vi "Periodic Tasks.vi"(8 "Error In":errorcluster) -> ()   [LabVIEW 2018]
doc: "This VI runs in parallel to other tasks. It can contain as many user-defined periodic loops as you need. These can carry out PID or other sorts of timed response."
uses:
  <vilib>/Rock Robotics/WPI/Solenoid/WPI_SolenoidValue.ctl
  <vilib>/Rock Robotics/WPI/ThirdParty/Phoenix-LabVIEW/Motor Controller/Controls/CTRE_Phoenix_MotorControl_ControlMode.ctl
  <vilib>/Rock Robotics/WPI/Utilities/WPI_GetSetVariantRefNum.vi
  Global 1.vi
  <vilib>/Rock Robotics/Network Tables/NT Write Boolean.vi
  <vilib>/Rock Robotics/Network Tables/NT Write Number.vi
  <vilib>/Rock Robotics/WPI/Solenoid/WPI_SolenoidSetEnum.vi
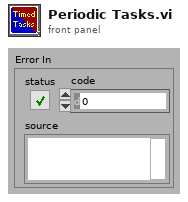
[diagram p1: front panel]
types:
  T1 = typedef "WPI_SwitchDevRef.ctl" = cluster{"DevStatus":errorcluster, "DIO Channel":T2, "CntIndex":T3, "Normally Closed":bool}
  T2 = typedef "FPGA_DIOChannel.ctl" = enum8{"DIO 0", "DIO 1", "DIO 2", "DIO 3", "DIO 4", "DIO 5", "DIO 6", "DIO 7", "DIO 8", "DIO 9", "DIO MXP 0", "DIO MXP 1", "DIO MXP 2", "DIO MXP 3", "DIO MXP 4", "DIO MXP 5", "DIO MXP 6", "DIO MXP 7", "DIO MXP 8", "DIO MXP 9", "DIO MXP 10", "DIO MXP 11", "DIO MXP 12", "DIO MXP 13", "DIO MXP 14", "DIO MXP 15", "SPI Port CS1", "SPI Port CS2", "SPI Port CS3", "SPI Port MISO", "SPI Port MOSI", "Invalid"}
  T3 = typedef "FPGA_CounterCtrSystemIndex.ctl" = enum8{"Ctr 0", "Ctr 1", "Ctr 2", "Ctr 3", "Ctr 4", "Ctr 5", "Ctr 6", "Ctr 7", "Invalid"}
  T4 = typedef "WPI_MotorControlDeviceRef.ctl" = cluster{"DeviceStatus":errorcluster, "Type":T5, "PWM":cluster{"PWM Channel":T6, "DeadBand":T7}, "CAN":cluster{"Device Number":u8, "SetOutput VI Ref":variant, "GetOutput VI Ref":variant, "Enable VI Ref":variant, "Disable VI Ref":variant, "Data":variant}, "Invert":bool, "DIO PWM":cluster{"PWM \"Enable\" Channel":T6, "DIOChannel":T2, "PWM Rate":dbl}}
  T5 = typedef "WPI_MotorControlType.ctl" = enum16{"PWM", "CAN", "DIO PWM"}
  T6 = typedef "FPGA_DIOPWMChannel.ctl" = enum8{"PWM 0", "PWM 1", "PWM 2", "PWM 3", "PWM 4", "PWM 5", "PWM 6", "PWM 7", "PWM 8", "PWM 9", "PWM MXP 0", "PWM MXP 1", "PWM MXP 2", "PWM MXP 3", "PWM MXP 4", "PWM MXP 5", "PWM MXP 6", "PWM MXP 7", "PWM MXP 8", "PWM MXP 9", "Invalid"}
  T7 = typedef "WPI_PWMDeadband.ctl" = cluster{"Name":string, "maxPositivePwm":i32, "minPositivePwm":i32, "centerPwm":i32, "maxNegativePwm":i32, "minNegativePwm":i32, "angularRange":u16}
  T8 = typedef "WPI_JoystickDevRef.ctl" = cluster{"Device":T9}
  T9 = typedef "WPI_JoystickDeviceEnum.ctl" = enum16{"USB 0", "USB 1", "USB 2", "USB 3", "USB 4", "USB 5"}
  T10 = typedef "CTRE_Phoenix_MotorControl_ControlMode.ctl" = u16
  T11 = typedef "WPI_SolenoidDevRef.ctl" = cluster{"DevStatus":errorcluster, "Pneumatics Control Module":u8, "Forward Solenoid Channel":T12, "Reverse Solenoid Channel":T12}
  T12 = typedef "WPI_SolenoidChannel.ctl" = enum8{"Solenoid 0", "Solenoid 1", "Solenoid 2", "Solenoid 3", "Solenoid 4", "Solenoid 5", "Solenoid 6", "Solenoid 7", "Invalid"}
  T13 = typedef "WPI_SolenoidValue.ctl" = enum16{"Off", "On", "Forward", "Reverse"}
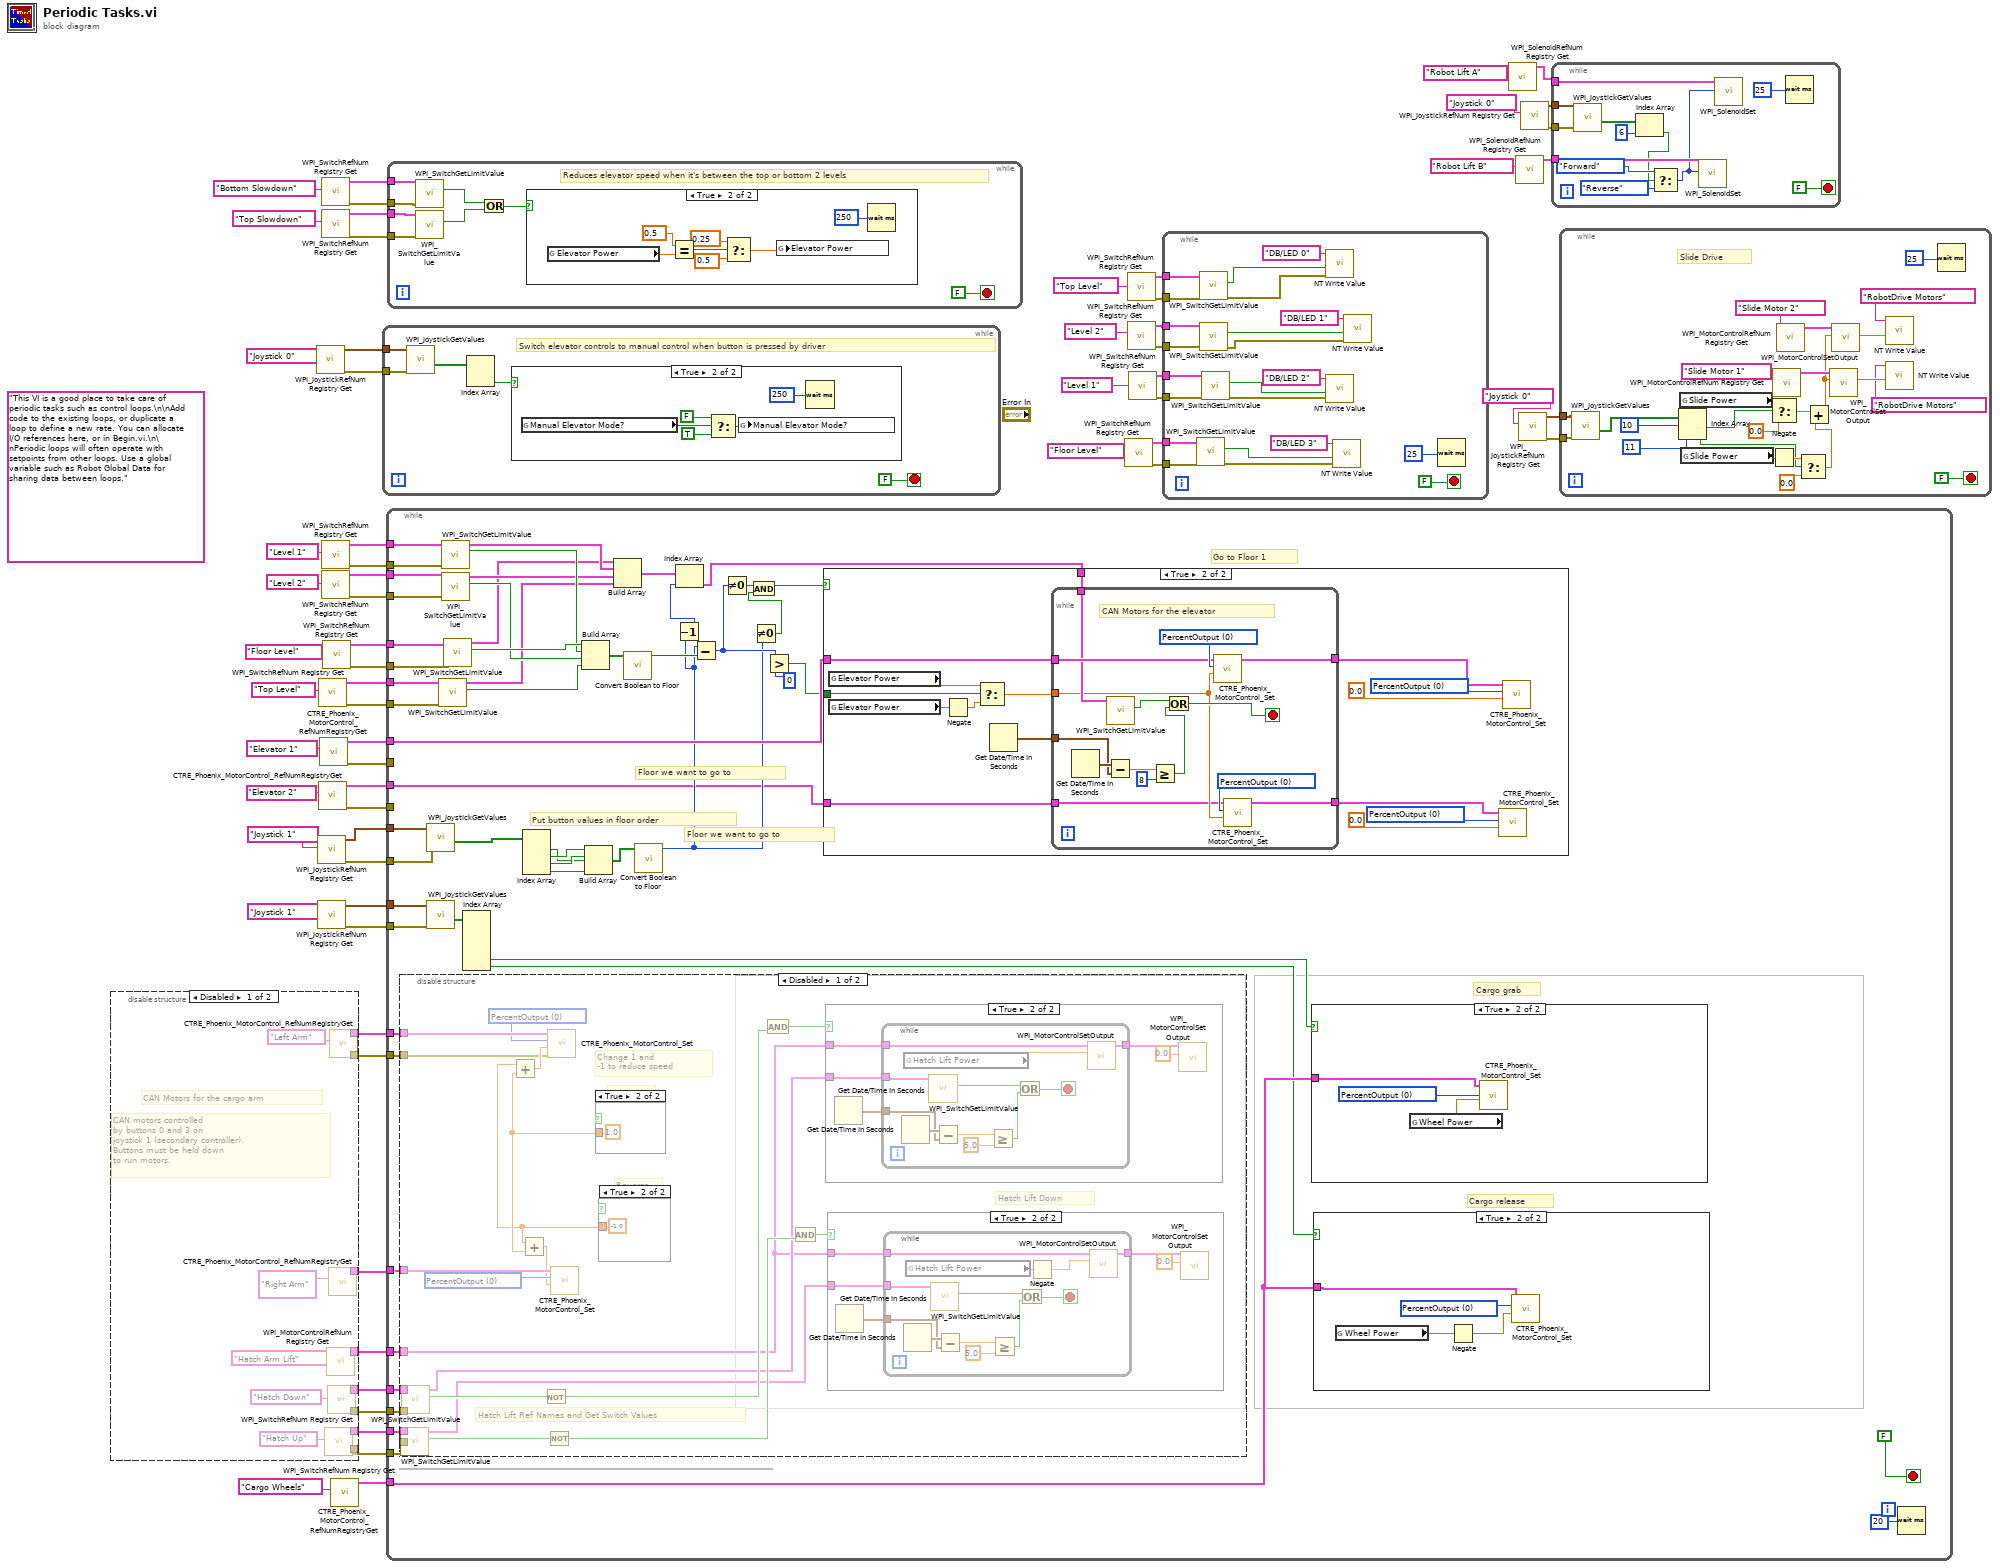
[diagram p0: block diagram]
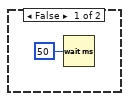
[diagram p3: hidden frame]
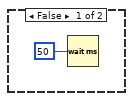
[diagram p4: hidden frame]
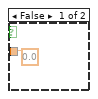
[diagram p7: hidden frame]
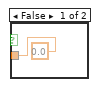
[diagram p8: hidden frame]
diagram:
  (unwired) "This VI is a good place to take care of periodic tasks such as control loops.\n\nAdd code to the existing loops, or duplicate a loop to define a new rate. You can allocate I/O references here, or in Begin.vi.\n\nPeriodic loops will often operate with setpoints from other loops. Use a global variable such as Robot Global Data for sharing data between loops."
  n1 = disable-structure shown="Disabled" {
    disable-tunnel: [w78 _] -> w63
    disable-tunnel: [w77 _] -> w62
    disable-tunnel: [w74 _] -> w46
    disable-tunnel: [w70 _] -> w33
    disable-tunnel: [w69 _] -> w32
    disable-tunnel: [w68 _] -> w31
    disable-tunnel: [w67 _] -> w30
    disable-tunnel: [w66 _] -> w29
    frame Disabled {
      # "CAN Motors for the cargo arm"
      # "CAN motors controlled\nby buttons 0 and 3 on \njoystick 1 (secondary controller).\nButtons must be held down\nto run motors."
      n2 = call <vilib>:"WPI_SwitchRefNum Registry Get.vi"("refnum name"="Hatch Up") -> ("error out"=w69:errorcluster, "SwitchDevRef"=w70:T1)  [unwired: 9 in]
      n3 = call <vilib>:"WPI_MotorControlRefNum Registry Get.vi"("refnum name"="Hatch Arm Lift") -> ("MotorControlDevRef"=w66:T4)  [unwired: 9 in, 1 out]
      n4 = call <vilib>:"WPI_SwitchRefNum Registry Get.vi"("refnum name"="Hatch Down") -> ("error out"=w68:errorcluster, "SwitchDevRef"=w67:T1)  [unwired: 9 in]
      n5 = call <vilib>:"CTRE_Phoenix_MotorControl_RefNumRegistryGet.vi"("refnum name"="Right Arm") -> ("PhoenixMotorControlDevRef"=w77:T4)  [unwired: 9 in, 1 out]
      n6 = call <vilib>:"CTRE_Phoenix_MotorControl_RefNumRegistryGet.vi"("refnum name"="Left Arm") -> ("error out"=w74:errorcluster, "PhoenixMotorControlDevRef"=w78:T4)  [unwired: 9 in]
    }
    frame Enabled {
    }
  }
  n7 = call <vilib>:"WPI_JoystickRefNum Registry Get.vi"("refnum name"="Joystick 0") -> ("error out"=w53:errorcluster, "JoystickDevRef"=w54:T8)  [unwired: 9 in]
  n8 = call <vilib>:"WPI_JoystickRefNum Registry Get.vi"("refnum name"="Joystick 1") -> ("error out"=w47:errorcluster, "JoystickDevRef"=w58:T8)  [unwired: 9 in]
  n9 = call <vilib>:"WPI_JoystickRefNum Registry Get.vi"("refnum name"="Joystick 1") -> ("error out"=w52:errorcluster, "JoystickDevRef"=w60:T8)  [unwired: 9 in]
  n10 = call <vilib>:"WPI_SwitchRefNum Registry Get.vi"("refnum name"="Top Level") -> ("error out"=w51:errorcluster, "SwitchDevRef"=w61:T1)  [unwired: 9 in]
  n11 = call <vilib>:"CTRE_Phoenix_MotorControl_RefNumRegistryGet.vi"("refnum name"="Elevator 2") -> ("error out"=w14:errorcluster, "PhoenixMotorControlDevRef"=w21:T4)  [unwired: 9 in]
  n12 = call <vilib>:"CTRE_Phoenix_MotorControl_RefNumRegistryGet.vi"("refnum name"="Elevator 1") -> ("error out"=w13:errorcluster, "PhoenixMotorControlDevRef"=w59:T4)  [unwired: 9 in]
  n13 = call <vilib>:"WPI_SwitchRefNum Registry Get.vi"("refnum name"="Bottom Slowdown") -> ("error out"=w15:errorcluster, "SwitchDevRef"=w18:T1)  [unwired: 9 in]
  n14 = call <vilib>:"WPI_SwitchRefNum Registry Get.vi"("refnum name"="Top Slowdown") -> ("error out"=w16:errorcluster, "SwitchDevRef"=w17:T1)  [unwired: 9 in]
  n15 = call <vilib>:"WPI_SwitchRefNum Registry Get.vi"("refnum name"="Level 1") -> ("error out"=w48:errorcluster, "SwitchDevRef"=w65:T1)  [unwired: 9 in]
  n16 = call <vilib>:"WPI_SwitchRefNum Registry Get.vi"("refnum name"="Level 2") -> ("error out"=w49:errorcluster, "SwitchDevRef"=w64:T1)  [unwired: 9 in]
  n17 = call <vilib>:"WPI_SwitchRefNum Registry Get.vi"("refnum name"="Floor Level") -> ("error out"=w50:errorcluster, "SwitchDevRef"=w57:T1)  [unwired: 9 in]
  n18 = call <vilib>:"CTRE_Phoenix_MotorControl_RefNumRegistryGet.vi"("refnum name"="Cargo Wheels") -> ("PhoenixMotorControlDevRef"=w3:T4)  [unwired: 9 in, 1 out]
  n19 = while {
    tunnel: w54 -> [w83]
    tunnel: w53 -> [w82]
    stop <- FALSE stop-if-true
    # "Switch elevator controls to manual control when button is pressed by driver"
    n20 = call <vilib>:"WPI_JoystickGetValues.vi"("error in (no error)"=w82, "JoystickDevRef"=w83) -> ("Buttons"=w81:bool[])  [unwired: 5 in, 4 out]
    n21 = Index Array(array=w81) -> (element #2=w80:bool)  [unwired: 2 in, 1 out]
    n22 = case shown="True" w80 {
      frame False {
        n23 = Wait (ms)(milliseconds to wait=u32 50) -> ()  [unwired: 1 out]
      }
      frame True {
        n24 = global read "Global 1.vi" "Manual Elevator Mode?"() -> (w89:bool)
        n25 = Select(t=FALSE, s=w89, f=TRUE) -> (s? t:f=w88:bool)
        n26 = global write "Global 1.vi" "Manual Elevator Mode?"(w88) -> ()
        n27 = Wait (ms)(milliseconds to wait=u32 250) -> ()  [unwired: 1 out]
      }
    }
  }
  n28 = while {
    tunnel: w65 -> [w141]
    tunnel: w64 -> [w140]
    tunnel: w63 -> [w139]
    tunnel: w62 -> [w138]
    tunnel: w61 -> [w137]
    tunnel: w60 -> [w136]
    tunnel: w59 -> [w133]
    tunnel: w58 -> [w135]
    tunnel: w57 -> [w134]
    tunnel: w52 -> [w131]
    tunnel: w51 -> [w130]
    tunnel: w50 -> [w129]
    tunnel: w49 -> [w128]
    tunnel: w48 -> [w127]
    tunnel: w47 -> [w126]
    tunnel: w46 -> [w125]
    tunnel: w33 -> [w124]
    tunnel: w32 -> [w123]
    tunnel: w31 -> [w122]
    tunnel: w30 -> [w121]
    tunnel: w29 -> [w120]
    tunnel: w3 -> [w119]
    tunnel: w21 -> [w98]
    tunnel: w14 -> [_]
    tunnel: w13 -> [_]
    stop <- FALSE stop-if-true
    # "Put button values in floor order"
    # "Floor we want to go to"
    # "Floor we want to go to"
    # "Go to Floor 1"
    # "Cargo release"
    # "Cargo grab"
    n29 = disable-structure shown="Disabled" {
      disable-tunnel: w139 -> [w165 _]
      disable-tunnel: w138 -> [w164 _]
      disable-tunnel: w125 -> [w157 _]
      disable-tunnel: w124 -> [w156 _]
      disable-tunnel: w123 -> [w155 _]
      disable-tunnel: w122 -> [w154 _]
      disable-tunnel: w121 -> [w153 _]
      disable-tunnel: w120 -> [w145 _]
      frame Disabled {
        w161 = T10 0 items=["PercentOutput"=0, "Position"=1, "Velocity"=2, "Current"=3, "Follower"=5, "MotionProfile"=6, "MotionMagic"=7, "MotionProfileArc"=10, "Disabled"=15] ("Control Mode")
        w163 = T10 0 items=["PercentOutput"=0, "Position"=1, "Velocity"=2, "Current"=3, "Follower"=5, "MotionProfile"=6, "MotionMagic"=7, "MotionProfileArc"=10, "Disabled"=15] ("Control Mode")
        # "Hatch Lift Ref Names and Get Switch Values"
        # "Hatch Lift Down"
        # "Change 1 and\n-1 to reduce speed"
        # "Forward"
        # "Reverse"
        n30 = call <vilib>:"WPI_SwitchGetLimitValue.vi"("error in (no error)"=w155, "SwitchDevRef"=w156) -> ("Switch Pressed"=w152:bool, "SwitchDevRef"=w144:T1)  [unwired: 7 in, 1 out]
        n31 = call <vilib>:"WPI_SwitchGetLimitValue.vi"("error in (no error)"=w154, "SwitchDevRef"=w153) -> ("Switch Pressed"=w150:bool, "SwitchDevRef"=w146:T1)  [unwired: 7 in, 1 out]
        n32 = Not(x=w150) -> (.not. x?=w149:bool)
        n33 = Not(x=w152) -> (.not. x?=w148:bool)
        n34 = case shown="True" {
          selector: _ -> [_ _]
          tunnel: [0.0 1.0] -> w159
          frame False {
          }
          frame True {
          }
        }
        n35 = case shown="True" {
          selector: _ -> [_ _]
          tunnel: [0.0 -1.0] -> w158
          frame False {
          }
          frame True {
          }
        }
        n36 = Add(x=w158, y=w159) -> (x+y=w162:dbl)
        n37 = Add(x=w158, y=w159) -> (x+y=w160:dbl)
        n38 = call <vilib>:"CTRE_Phoenix_MotorControl_Set.vi"("error in (no error)"=w157, "Output"=w162, "Control Mode"=w163, "PhoenixMotorControlDevRef"=w165) -> ()  [unwired: 6 in, 2 out]
        n39 = call <vilib>:"CTRE_Phoenix_MotorControl_Set.vi"("Output"=w160, "Control Mode"=w161, "PhoenixMotorControlDevRef"=w164) -> ()  [unwired: 7 in, 2 out]
        n40 = And(y=w149) -> (x .and. y?=w151:bool)  [unwired: 1 in]
        n41 = And(y=w148) -> (x .and. y?=w147:bool)  [unwired: 1 in]
        n42 = case shown="True" w151 {
          tunnel: w146 -> [_ w187]
          tunnel: w145 -> [_ w186]
          frame False {
          }
          frame True {
            n43 = Get Date/Time In Seconds() -> (seconds since 1Jan1904=w185:timestamp)
            n44 = while {
              tunnel: w187 -> [w198]
              tunnel: w186 -> [w197]
              tunnel: w185 -> [w193]
              tunnel: [w189] -> w184
              stop <- w192 stop-if-true
              n45 = Get Date/Time In Seconds() -> (seconds since 1Jan1904=w194:timestamp)
              n46 = global read "Global 1.vi" "Hatch Lift Power"() -> (w196:dbl)
              n47 = call <vilib>:"WPI_SwitchGetLimitValue.vi"("SwitchDevRef"=w198) -> ("Switch Pressed"=w191:bool)  [unwired: 8 in, 2 out]
              n48 = Subtract(x=w194, y=w193) -> (x-y=w195:dbl)
              n49 = Greater Or Equal?(x=w195, y=5.0) -> (x >= y?=w190:bool)
              n50 = Or(x=w191, y=w190) -> (x .or. y?=w192:bool)
              n51 = call <vilib>:"WPI_MotorControlSetOutput.vi"("Output"=w196, "MotorControlDevRef"=w197) -> ("MotorControlDevRef"=w189:T4)  [unwired: 7 in, 2 out]
            }
            n52 = call <vilib>:"WPI_MotorControlSetOutput.vi"("Output"=0.0, "MotorControlDevRef"=w184) -> ()  [unwired: 7 in, 3 out]
          }
        }
        n53 = case shown="True" w147 {
          tunnel: w144 -> [_ w170]
          tunnel: w145 -> [_ w169]
          frame False {
          }
          frame True {
            n54 = Get Date/Time In Seconds() -> (seconds since 1Jan1904=w168:timestamp)
            n55 = while {
              tunnel: w170 -> [w182]
              tunnel: w169 -> [w181]
              tunnel: w168 -> [w177]
              tunnel: [w173] -> w167
              stop <- w176 stop-if-true
              n56 = Get Date/Time In Seconds() -> (seconds since 1Jan1904=w178:timestamp)
              n57 = global read "Global 1.vi" "Hatch Lift Power"() -> (w180:dbl)
              n58 = call <vilib>:"WPI_SwitchGetLimitValue.vi"("SwitchDevRef"=w182) -> ("Switch Pressed"=w175:bool)  [unwired: 8 in, 2 out]
              n59 = Subtract(x=w178, y=w177) -> (x-y=w179:dbl)
              n60 = Greater Or Equal?(x=w179, y=5.0) -> (x >= y?=w174:bool)
              n61 = Or(x=w175, y=w174) -> (x .or. y?=w176:bool)
              n62 = Negate(x=w180) -> (-x=w172:dbl)
              n63 = call <vilib>:"WPI_MotorControlSetOutput.vi"("Output"=w172, "MotorControlDevRef"=w181) -> ("MotorControlDevRef"=w173:T4)  [unwired: 7 in, 2 out]
            }
            n64 = call <vilib>:"WPI_MotorControlSetOutput.vi"("Output"=0.0, "MotorControlDevRef"=w167) -> ()  [unwired: 7 in, 3 out]
          }
        }
      }
      frame Enabled {
      }
    }
    n65 = call <vilib>:"WPI_JoystickGetValues.vi"("error in (no error)"=w126, "JoystickDevRef"=w135) -> ("Buttons"=w97:bool[])  [unwired: 5 in, 4 out]
    n66 = call <vilib>:"WPI_JoystickGetValues.vi"("error in (no error)"=w131, "JoystickDevRef"=w136) -> ("Buttons"=w132:bool[])  [unwired: 5 in, 4 out]
    n67 = call <vilib>:"WPI_SwitchGetLimitValue.vi"("error in (no error)"=w130, "SwitchDevRef"=w137) -> ("Switch Pressed"=w117:bool, "SwitchDevRef"=w106:T1)  [unwired: 7 in, 1 out]
    n68 = call <vilib>:"WPI_SwitchGetLimitValue.vi"("error in (no error)"=w127, "SwitchDevRef"=w141) -> ("Switch Pressed"=w115:bool, "SwitchDevRef"=w108:T1)  [unwired: 7 in, 1 out]
    n69 = call <vilib>:"WPI_SwitchGetLimitValue.vi"("error in (no error)"=w128, "SwitchDevRef"=w140) -> ("Switch Pressed"=w114:bool, "SwitchDevRef"=w107:T1)  [unwired: 7 in, 1 out]
    n70 = call <vilib>:"WPI_SwitchGetLimitValue.vi"("error in (no error)"=w129, "SwitchDevRef"=w134) -> ("Switch Pressed"=w116:bool, "SwitchDevRef"=w105:T1)  [unwired: 7 in, 1 out]
    n71 = Index Array(array=w132) -> (element #5=w91:bool, element #6=w90:bool)  [unwired: 6 in, 4 out]
    n72 = Index Array(array=w97) -> (element #1=w94:bool, element #2=w96:bool, element #3=w95:bool, element #4=w93:bool)  [unwired: 4 in]
    n73 = Build Array(w116, w115, w114, w117) -> (w118:bool[])
    n74 = Build Array(w96, w95, w94, w93) -> (w92:bool[])
    n75 = Build Array(w105, w108, w107, w106) -> (w104:T1[])
    n76 = call "Convert Boolean to Floor.vi"("Boolean array"=w118) -> ("Floor Number"=w112:i32)  [unwired: 8 in, 2 out]
    n77 = call "Convert Boolean to Floor.vi"("Boolean array"=w92) -> ("Floor Number"=w100:i32)  [unwired: 8 in, 2 out]
    n78 = Decrement(x=w100) -> (x-1=w102:i32)
    n79 = Index Array(array=w104, index=w102) -> (element=w103:T1)
    n80 = Subtract(x=w100, y=w112) -> (x-y=w111:i32)
    n81 = Not Equal To 0?(x=w111) -> (x != 0?=w113:bool)
    n82 = Not Equal To 0?(x=w100) -> (x != 0?=w99:bool)
    n83 = And(x=w113, y=w99) -> (x .and. y?=w101:bool)
    n84 = Greater?(x=w111, y=0) -> (0:w109:bool)
    n85 = case shown="True" w101 {
      tunnel: w133 -> [_ w217]
      tunnel: w103 -> [_ w213]
      tunnel: w109 -> [_ w210]
      tunnel: w98 -> [_ w203]
      frame False {
      }
      frame True {
        w206 = T10 0 items=["PercentOutput"=0, "Position"=1, "Velocity"=2, "Current"=3, "Follower"=5, "MotionProfile"=6, "MotionMagic"=7, "MotionProfileArc"=10, "Disabled"=15] ("Control Mode")
        w216 = T10 0 items=["PercentOutput"=0, "Position"=1, "Velocity"=2, "Current"=3, "Follower"=5, "MotionProfile"=6, "MotionMagic"=7, "MotionProfileArc"=10, "Disabled"=15] ("Control Mode")
        n86 = global read "Global 1.vi" "Elevator Power"() -> (w209:dbl)
        n87 = global read "Global 1.vi" "Elevator Power"() -> (w207:dbl)
        n88 = Negate(x=w207) -> (-x=w208:dbl)
        n89 = Select(t=w209, s=w210, f=w208) -> (s? t:f=w212:dbl)
        n90 = Get Date/Time In Seconds() -> (seconds since 1Jan1904=w211:timestamp)
        n91 = while {
          tunnel: w217 -> [w231]
          tunnel: [w230] -> w214
          tunnel: w213 -> [w229]
          tunnel: w212 -> [w221]
          tunnel: w211 -> [w225]
          tunnel: [w219] -> w205
          tunnel: w203 -> [w218]
          stop <- w228 stop-if-true
          w220 = T10 0 items=["PercentOutput"=0, "Position"=1, "Velocity"=2, "Current"=3, "Follower"=5, "MotionProfile"=6, "MotionMagic"=7, "MotionProfileArc"=10, "Disabled"=15] ("Control Mode")
          w232 = T10 0 items=["PercentOutput"=0, "Position"=1, "Velocity"=2, "Current"=3, "Follower"=5, "MotionProfile"=6, "MotionMagic"=7, "MotionProfileArc"=10, "Disabled"=15] ("Control Mode")
          # "CAN Motors for the elevator"
          n92 = Get Date/Time In Seconds() -> (seconds since 1Jan1904=w226:timestamp)
          n93 = call <vilib>:"WPI_SwitchGetLimitValue.vi"("SwitchDevRef"=w229) -> ("Switch Pressed"=w227:bool)  [unwired: 8 in, 2 out]
          n94 = Subtract(x=w226, y=w225) -> (x-y=w223:dbl)
          n95 = Greater Or Equal?(x=w223, y=8) -> (x >= y?=w222:bool)
          n96 = Or(x=w227, y=w222) -> (x .or. y?=w228:bool)
          n97 = call <vilib>:"CTRE_Phoenix_MotorControl_Set.vi"("Output"=w221, "Control Mode"=w232, "PhoenixMotorControlDevRef"=w231) -> ("PhoenixMotorControlDevRef"=w230:T4)  [unwired: 7 in, 1 out]
          n98 = call <vilib>:"CTRE_Phoenix_MotorControl_Set.vi"("Output"=w221, "Control Mode"=w220, "PhoenixMotorControlDevRef"=w218) -> ("PhoenixMotorControlDevRef"=w219:T4)  [unwired: 7 in, 1 out]
        }
        n99 = call <vilib>:"CTRE_Phoenix_MotorControl_Set.vi"("Output"=0.0, "Control Mode"=w206, "PhoenixMotorControlDevRef"=w205) -> ()  [unwired: 7 in, 2 out]
        n100 = call <vilib>:"CTRE_Phoenix_MotorControl_Set.vi"("Output"=0.0, "Control Mode"=w216, "PhoenixMotorControlDevRef"=w214) -> ()  [unwired: 7 in, 2 out]
      }
    }
    n101 = case shown="True" w91 {
      tunnel: w119 -> [_ w237]
      frame False {
      }
      frame True {
        w238 = T10 0 items=["PercentOutput"=0, "Position"=1, "Velocity"=2, "Current"=3, "Follower"=5, "MotionProfile"=6, "MotionMagic"=7, "MotionProfileArc"=10, "Disabled"=15] ("Control Mode")
        n102 = global read "Global 1.vi" "Wheel Power"() -> (w239:dbl)
        n103 = call <vilib>:"CTRE_Phoenix_MotorControl_Set.vi"("Output"=w239, "Control Mode"=w238, "PhoenixMotorControlDevRef"=w237) -> ()  [unwired: 7 in, 2 out]
      }
    }
    n104 = case shown="True" w90 {
      tunnel: w119 -> [_ w235]
      frame False {
      }
      frame True {
        w236 = T10 0 items=["PercentOutput"=0, "Position"=1, "Velocity"=2, "Current"=3, "Follower"=5, "MotionProfile"=6, "MotionMagic"=7, "MotionProfileArc"=10, "Disabled"=15] ("Control Mode")
        n105 = global read "Global 1.vi" "Wheel Power"() -> (w234:dbl)
        n106 = Negate(x=w234) -> (-x=w233:dbl)
        n107 = call <vilib>:"CTRE_Phoenix_MotorControl_Set.vi"("Output"=w233, "Control Mode"=w236, "PhoenixMotorControlDevRef"=w235) -> ()  [unwired: 7 in, 2 out]
      }
    }
    n108 = Wait (ms)(milliseconds to wait=u32 20) -> ()  [unwired: 1 out]
  }
  n109 = while {
    tunnel: w18 -> [w247]
    tunnel: w17 -> [w246]
    tunnel: w16 -> [w245]
    tunnel: w15 -> [w244]
    stop <- FALSE stop-if-true
    # "Reduces elevator speed when it's between the top or bottom 2 levels"
    n110 = call <vilib>:"WPI_SwitchGetLimitValue.vi"("error in (no error)"=w244, "SwitchDevRef"=w247) -> ("Switch Pressed"=w243:bool)  [unwired: 7 in, 2 out]
    n111 = call <vilib>:"WPI_SwitchGetLimitValue.vi"("error in (no error)"=w245, "SwitchDevRef"=w246) -> ("Switch Pressed"=w241:bool)  [unwired: 7 in, 2 out]
    n112 = Or(x=w243, y=w241) -> (x .or. y?=w242:bool)
    n113 = case shown="True" w242 {
      frame False {
        n114 = Wait (ms)(milliseconds to wait=u32 50) -> ()  [unwired: 1 out]
      }
      frame True {
        n115 = global read "Global 1.vi" "Elevator Power"() -> (w255:dbl)
        n116 = Equal?(x=0.5, y=w255) -> (x = y?=w254:bool)
        n117 = Select(t=0.25, s=w254, f=0.5) -> (s? t:f=w250:dbl)
        n118 = global write "Global 1.vi" "Elevator Power"(w250) -> ()
        n119 = Wait (ms)(milliseconds to wait=u32 250) -> ()  [unwired: 1 out]
      }
    }
  }
  n120 = call <vilib>:"WPI_SwitchRefNum Registry Get.vi"("refnum name"="Floor Level") -> ("error out"=w40:errorcluster, "SwitchDevRef"=w39:T1)  [unwired: 9 in]
  n121 = call <vilib>:"WPI_SwitchRefNum Registry Get.vi"("refnum name"="Top Level") -> ("error out"=w44:errorcluster, "SwitchDevRef"=w45:T1)  [unwired: 9 in]
  n122 = call <vilib>:"WPI_SwitchRefNum Registry Get.vi"("refnum name"="Level 2") -> ("error out"=w42:errorcluster, "SwitchDevRef"=w43:T1)  [unwired: 9 in]
  n123 = call <vilib>:"WPI_SwitchRefNum Registry Get.vi"("refnum name"="Level 1") -> ("error out"=w38:errorcluster, "SwitchDevRef"=w41:T1)  [unwired: 9 in]
  n124 = while {
    tunnel: w45 -> [w277]
    tunnel: w44 -> [w276]
    tunnel: w43 -> [w275]
    tunnel: w42 -> [w274]
    tunnel: w41 -> [w273]
    tunnel: w40 -> [w272]
    tunnel: w39 -> [w271]
    tunnel: w38 -> [w270]
    stop <- FALSE stop-if-true
    n125 = call <vilib>:"WPI_SwitchGetLimitValue.vi"("error in (no error)"=w272, "SwitchDevRef"=w271) -> ("error out"=w256:errorcluster, "Switch Pressed"=w262:bool)  [unwired: 7 in, 1 out]
    n126 = call <vilib>:"WPI_SwitchGetLimitValue.vi"("error in (no error)"=w276, "SwitchDevRef"=w277) -> ("error out"=w259:errorcluster, "Switch Pressed"=w268:bool)  [unwired: 7 in, 1 out]
    n127 = call <vilib>:"WPI_SwitchGetLimitValue.vi"("error in (no error)"=w274, "SwitchDevRef"=w275) -> ("error out"=w258:errorcluster, "Switch Pressed"=w266:bool)  [unwired: 7 in, 1 out]
    n128 = call <vilib>:"WPI_SwitchGetLimitValue.vi"("error in (no error)"=w270, "SwitchDevRef"=w273) -> ("error out"=w257:errorcluster, "Switch Pressed"=w264:bool)  [unwired: 7 in, 1 out]
    n129 = call-poly <vilib>:"NT Write Value.vi"("error in"=w259, "Boolean"=w268, "Name"="DB/LED 0") -> ()  [unwired: 8 in, 1 out]
    n130 = call-poly <vilib>:"NT Write Value.vi"("error in"=w257, "Boolean"=w264, "Name"="DB/LED 2") -> ()  [unwired: 8 in, 1 out]
    n131 = call-poly <vilib>:"NT Write Value.vi"("error in"=w256, "Boolean"=w262, "Name"="DB/LED 3") -> ()  [unwired: 8 in, 1 out]
    n132 = call-poly <vilib>:"NT Write Value.vi"("error in"=w258, "Boolean"=w266, "Name"="DB/LED 1") -> ()  [unwired: 8 in, 1 out]
    n133 = Wait (ms)(milliseconds to wait=u32 25 ("millisecond timer value")) -> ()  [unwired: 1 out]
  }
  n134 = call <vilib>:"WPI_SolenoidRefNum Registry Get.vi"("refnum name"="Robot Lift A") -> ("SolenoidDevRef"=w1:T11)  [unwired: 9 in, 1 out]
  n135 = call <vilib>:"WPI_SolenoidRefNum Registry Get.vi"("refnum name"="Robot Lift B") -> ("SolenoidDevRef"=w5:T11)  [unwired: 9 in, 1 out]
  n136 = call <vilib>:"WPI_JoystickRefNum Registry Get.vi"("refnum name"="Joystick 0") -> ("error out"=w10:errorcluster, "JoystickDevRef"=w11:T8)  [unwired: 9 in]
  n137 = call <vilib>:"WPI_JoystickRefNum Registry Get.vi"("refnum name"="Joystick 0") -> ("error out"=w7:errorcluster, "JoystickDevRef"=w8:T8)  [unwired: 9 in]
  n138 = while {
    tunnel: w8 -> [w287]
    tunnel: w7 -> [w286]
    tunnel: w5 -> [w283]
    tunnel: w1 -> [w279]
    stop <- FALSE stop-if-true
    n139 = call <vilib>:"WPI_JoystickGetValues.vi"("error in (no error)"=w286, "JoystickDevRef"=w287) -> ("Buttons"=w285:bool[])  [unwired: 5 in, 4 out]
    n140 = Index Array(array=w285, index=6) -> (element=w280:bool)
    n141 = Select(t=WPI_SolenoidValue."Forward" ("Value"), s=w280, f=WPI_SolenoidValue."Reverse" ("Value")) -> (s? t:f=w278:T13)
    n142 = call-poly <vilib>:"WPI_SolenoidSet.vi"("Value"=w278, "SolenoidDevRef"=w283) -> ()  [unwired: 8 in, 2 out]
    n143 = call-poly <vilib>:"WPI_SolenoidSet.vi"("Value"=w278, "SolenoidDevRef"=w279) -> ()  [unwired: 8 in, 2 out]
    n144 = Wait (ms)(milliseconds to wait=u32 25 ("millisecond timer value")) -> ()  [unwired: 1 out]
  }
  n145 = while {
    tunnel: w11 -> [w296]
    tunnel: w10 -> [w295]
    stop <- FALSE stop-if-true
    # "Slide Drive"
    n146 = call <vilib>:"WPI_JoystickGetValues.vi"("error in (no error)"=w295, "JoystickDevRef"=w296) -> ("Buttons"=w297:bool[])  [unwired: 5 in, 4 out]
    n147 = Index Array(array=w297, index #1=10 ("index"), index #2=11 ("index")) -> (element #1=w292:bool, element #2=w291:bool)
    n148 = global read "Global 1.vi" "Slide Power"() -> (w305:dbl)
    n149 = global read "Global 1.vi" "Slide Power"() -> (w303:dbl)
    n150 = Select(t=w305, s=w292, f=0.0) -> (s? t:f=w300:dbl)
    n151 = Negate(x=w303) -> (-x=w302:dbl)
    n152 = call <vilib>:"WPI_MotorControlRefNum Registry Get.vi"("refnum name"="Slide Motor 1") -> ("MotorControlDevRef"=w313:T4)  [unwired: 9 in, 1 out]
    n153 = call <vilib>:"WPI_MotorControlRefNum Registry Get.vi"("refnum name"="Slide Motor 2") -> ("MotorControlDevRef"=w309:T4)  [unwired: 9 in, 1 out]
    n154 = Select(t=w302, s=w291, f=0.0) -> (s? t:f=w299:dbl)
    n155 = Add(x=w300, y=w299) -> (x+y=w301:dbl)
    n156 = call <vilib>:"WPI_MotorControlSetOutput.vi"("Output"=w301, "MotorControlDevRef"=w313) -> ("Motor Output"=w312:dbl)  [unwired: 7 in, 2 out]
    n157 = call <vilib>:"WPI_MotorControlSetOutput.vi"("Output"=w301, "MotorControlDevRef"=w309) -> ("Motor Output"=w307:dbl)  [unwired: 7 in, 2 out]
    n158 = call-poly <vilib>:"NT Write Value.vi"("Numeric"=w307, "Name"="RobotDrive Motors" ("refnum name")) -> ()  [unwired: 9 in, 1 out]
    n159 = call-poly <vilib>:"NT Write Value.vi"("Numeric"=w312, "Name"="RobotDrive Motors" ("refnum name")) -> ()  [unwired: 9 in, 1 out]
    n160 = Wait (ms)(milliseconds to wait=u32 25 ("millisecond timer value")) -> ()  [unwired: 1 out]
  }
